vi "emi_Ring from int arr.vi"(5 "Pre string(\"\")":string, 7 "Integer Array":i32[](array[numeric]), 9 "Disp / Val offset(0)":i32, 11 "error in (no error)":errorcluster) -> (8 "Ring selector":cluster{"String":string, "Value":dbl}[](array[cluster]), 15 "error out":errorcluster)   [LabVIEW 2010]
doc: "Creates a ring string and value array based on an integer array. This array can be written into a ring prperty node.\n\nDisp / Val offset. This value is added to the display, as compared to teh value.\n\nOn error: Create array as normals"
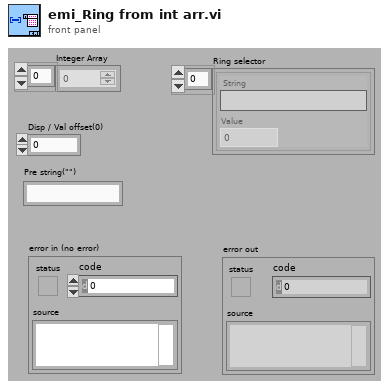
[diagram p1: front panel]
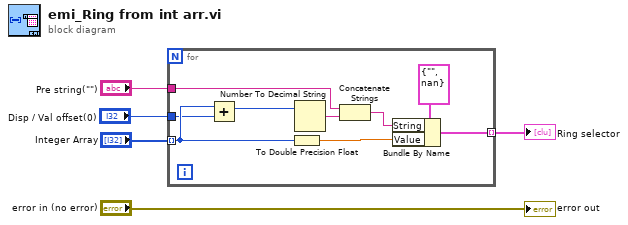
[diagram p0: block diagram]
diagram:
  n1 = for {
    tunnel: "Integer Array" -> [w12] mode=indexing
    tunnel: [w10] -> w5 mode=indexing
    tunnel: "Pre string(\"\")" -> [w8]
    tunnel: "Disp / Val offset(0)" -> [w6]
    n2 = Add(x=w12, y=w6) -> (x+y=w7:i32)
    n3 = To Double Precision Float(number=w12) -> (double precision float=w11:dbl)
    n4 = Number To Decimal String(number=w7) -> (decimal integer string=w13:string)  [unwired: 1 in]
    n5 = Concatenate Strings(w8, w13) -> (w9:string)
    n6 = Bundle By Name(cluster=cluster{"String":string, "Value":dbl} {"String"="", "Value"=nan}, "String"=w9, "Value"=w11) -> (w10:cluster{"String":string, "Value":dbl})
  }
  "Ring selector" <- w5
  "error out" <- "error in (no error)"
